vi "solar_voy Create.vi"(6 "Suppress Errors? (T)":bool=TRUE, 8 "error in (no error)":errorcluster, 9 "Create if not found? (T)":bool=TRUE, 10 "Setup":T1, 11 "Interface Name":string) -> (0 "error out":errorcluster, 1 "Created New?":bool, 3 "Voyager Refnum":T2)   [LabVIEW 2018]
doc: "This creates a Voyager reference and initializes the TCP header information."
uses:
  solar_voy_ctl Voyager Refnum.ctl
  solar_voy_ctl Setup.ctl
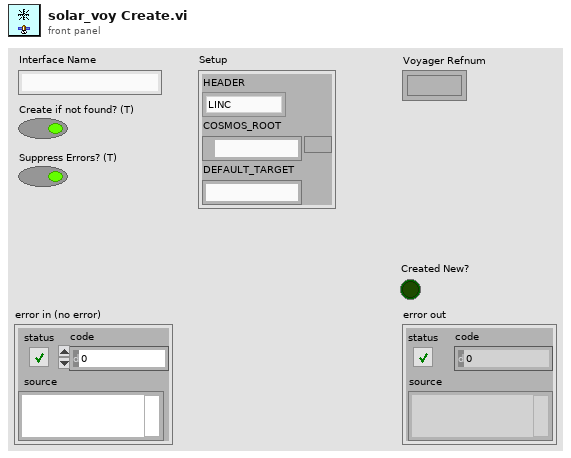
[diagram p1: front panel]
types:
  T1 = typedef "solar_voy_ctl Setup.ctl" = cluster{"HEADER":enum8{"LINC", "CCSDS"}, "COSMOS_ROOT":path, "DEFAULT_TARGET":string}
  T2 = typedef "solar_voy_ctl Voyager Refnum.ctl" = refnum<k1>
  T3 = typedef "solar_voy_def_ctl HDR.ctl" = cluster{"ITEMS":T4[], "LENGTH_NAME":string, "LENGTH_VALUE_OFFSET":i32, "ID_NAME":string, "ENDIAN":enum8{"BIG", "LITTLE"}, "GUID_NAME":string, "DEFAULT_TARGET":string, "DEFAULT_PACKET":string, "DEFAULT_ERROR":string}
  T4 = typedef "solar_voy_def_ctl ITEM.ctl" = cluster{"NAME":string, "OFFSET":i32, "SIZE":i32, "TYPE":T5, "EACH_SIZE":i32, "LVTYPE":T6, "MIN":dbl, "MAX":dbl, "DEFAULT":string, "DESC":string, "ID":bool, "MODIFIERS":variant, "last_value":variant}
  T5 = typedef "solar_voy_def_ctl ITEM TYPE.ctl" = enum8{"BLOCK", "INT", "UINT", "FLOAT", "STRING"}
  T6 = typedef "solar_type Item Type.ctl" = enum16{"NULL", "UNKNOWN", "CLUSTER", "I8", "I16", "I32", "I64", "U8", "U16", "U32", "U64", "U8_ENUM", "U16_ENUM", "U32_ENUM", "SGL", "DBL", "BOOLEAN", "STRING", "PATH", "VISA", "TAG", "TIME", "I8_1D", "I16_1D", "I32_1D", "I64_1D", "U8_1D", "U16_1D", "U32_1D", "U64_1D", "U8_ENUM_1D", "U16_ENUM_1D", "U32_ENUM_1D", "SGL_1D", "DBL_1D", "BOOLEAN_1D", "STRING_1D", "PATH_1D", "VISA_1D", "TAG_1D", "TIME_1D", "I8_2D", "I16_2D", "I32_2D", "I64_2D", "U8_2D", "U16_2D", "U32_2D", "U64_2D", "U8_ENUM_2D", "U16_ENUM_2D", "U32_ENUM_2D", "SGL_2D", "DBL_2D", "BOOLEAN_2D", "STRING_2D", "PATH_2D", "VISA_2D", "TAG_2D", "TIME_2D"}
  T7 = typedef "solar_voy_ctl Voyager.ctl" = cluster{"PACKETS":T8[], "COSMOS_Root":path, "CMD_HDR":T3, "TLM_HDR":T3, "TCPs":T10[], "VoyagerIDOffset":cluster{"VoyagerIDOffset":u16[], "Target Names":string[]}}
  T8 = typedef "solar_voy_def_ctl PACKET.ctl" = cluster{"PACKET_ID":T9, "ENDIAN":enum8{"BIG", "LITTLE"}, "DESC":string, "HZRD":bool, "ITEMS":T4[], "NoExport":bool, "last_time":timestamp, "last_count":u32, "last_data":string}
  T9 = typedef "solar_voy_def_ctl PACKET_ID.ctl" = cluster{"ID":u16, "CMD":enum8{"CMD", "TLM"}, "TARGET":string, "PACKET":string}
  T10 = typedef "solar_voy_ctl TCP.ctl" = cluster{"Connected":bool, "Port":u16, "Listener":refnum<k5>, "ServerIP":string, "TCP":refnum<k5>, "Setup":T11, "VIRefnum":refnum<vi>, "TARGETS_CMD":string[], "TARGETS_TLM":string[]}
  T11 = typedef "solar_voy_ctl Port Setup.ctl" = enum8{"SERVER", "CLIENT", "SERVER_CMD", "SERVER_TLM"}
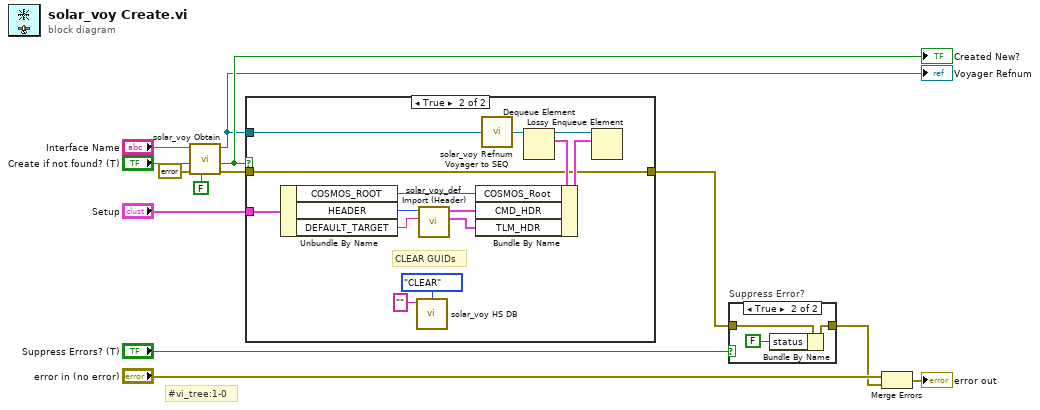
[diagram p0: block diagram]
diagram:
  # "#vi_tree:1-0"
  n1 = call "solar_voy Obtain.vi"("Suppress Errors? (T)"=FALSE, "error in (no error)"=errorcluster {"status"=FALSE, "code"=0, "source"=""}, "Create if not found? (T)"="Create if not found? (T)", "Interface Name"="Interface Name") -> ("error out"=w5:errorcluster, "Created New?"=w4:bool, "Voyager Refnum"=w2:T2)  [unwired: 5 in]
  "Voyager Refnum" <- w2
  "Created New?" <- w4
  n2 = case shown="True" w4 {
    tunnel: [w14 w22] -> w1
    tunnel: w5 -> [w14 w22]
    tunnel: w2 -> [_ w27]
    tunnel: "Setup" -> [_ w28]
    frame False {
    }
    frame True {
      # "CLEAR GUIDs"
      n3 = Unbundle By Name(w28) -> ("COSMOS_ROOT"=w21:path, "HEADER"=w18:enum8{"LINC", "CCSDS"}, "DEFAULT_TARGET"=w17:string)
      n4 = call "solar_voy HS DB.vi"("HDR_GUID"="", "Action"=enum8{"DELETE", "ADD", "CLEAR"}."CLEAR") -> ()  [unwired: 9 in, 5 out]
      n5 = call "solar_voy_def Import (Header).vi"("DEFAULT_TARGET"=w17, "HEADER"=w18) -> ("TLM_HDR"=w19:T3, "CMD_HDR"=w20:T3)  [unwired: 8 in]
      n6 = call "solar_voy Refnum Voyager to SEQ.vi"("Voyager Refnum"=w27) -> ("Voyager SEQ"=w26:refnum<queue>)
      n7 = Dequeue Element(queue=w26) -> (queue out=w25:refnum<queue>, element=w24:T7)  [unwired: 2 in, 2 out]
      n8 = Bundle By Name(cluster=w24, "COSMOS_Root"=w21, "CMD_HDR"=w20, "TLM_HDR"=w19) -> (w23:T7)
      n9 = Lossy Enqueue Element(queue=w25, element=w23) -> ()  [unwired: 1 in, 4 out]
    }
  }
  n10 = case "Suppress Error?" shown="True" "Suppress Errors? (T)" {
    tunnel: w1 -> [w29 w32]
    tunnel: [w29 w31] -> w7
    frame False {
    }
    frame True {
      n11 = Bundle By Name(cluster=w32, "status"=FALSE) -> (w31:errorcluster)
    }
  }
  n12 = Merge Errors("error in (no error)", w7) -> (→"error out":errorcluster)
